vi "testUnflattenForceFromXML.vi"() -> ()   [LabVIEW 2012, in "UnitsAndXML.lvlib"]
uses:
  <userlib>/Common/UnitsAndXML/UnitsAndXML.lvlib
  <userlib>/Common/UnitsAndXML/FlattenItemWithUnitToXML/FlattenForceToXML/ForceUnit.ctl
  <userlib>/Common/UnitsAndXML/UnflattenItemWithUnitFromXML/UnflattenForceFromXML/typeMethods/unflattenForceFromXML_Array.vi
  <userlib>/Common/UnitsAndXML/UnflattenItemWithUnitFromXML/UnflattenForceFromXML/typeMethods/unflattenForceFromXML_Scalar.vi
panel:
  out "error out":errorcluster
  out "force":dbl[unit][](array[numeric])
  out "force":dbl[unit]
  in  "forceUnitInXML":T1
  in  "xmlStringArray":string="<force>15</force>\r\n<force>30</force>\r\n<force>45</force>\r\n<force>60</force>"
  in  "xmlStringScalar":string="<force>15</force>"
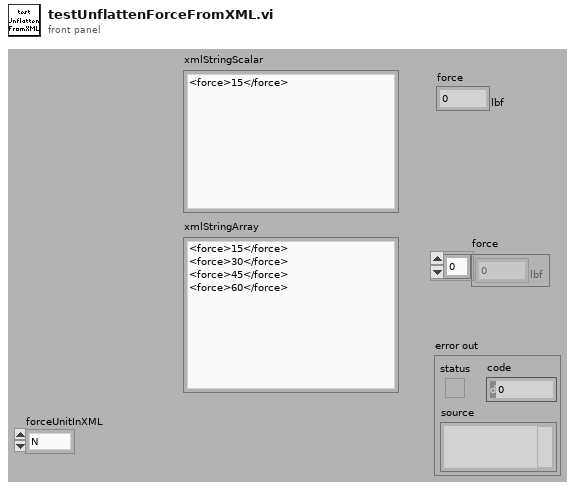
[diagram p1: front panel]
types:
  T1 = typedef "UnitsAndXML.lvlib/ForceUnit.ctl" = enum16{"N", "dyn", "lbf"}
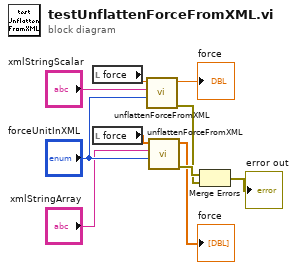
[diagram p0: block diagram]
diagram:
  n1 = local read "force"() -> (w10:dbl[unit])
  n2 = local read "force"() -> (w4:dbl[unit][])
  n3 = call-poly <userlib>:"unflattenForceFromXML.vi"("forceUnitInXML"="forceUnitInXML", "xmlString"="xmlStringScalar", "forceForType"=w10) -> ("error out"=w8:errorcluster, "force"=→"force":dbl[unit])  [unwired: 7 in]
  n4 = call-poly <userlib>:"unflattenForceFromXML.vi"("forceUnitInXML"="forceUnitInXML", "xmlString"="xmlStringArray", "forceForType"=w4) -> ("error out"=w9:errorcluster, "force"=→"force":dbl[unit][])  [unwired: 7 in]
  n5 = Merge Errors(w9, w8) -> (→"error out":errorcluster)
